vi "Enabled Channel Mask To Number.vi"(0 "selected acquisition channels to store":bool[](array[boolean])) -> (4 "number of selected channels":u8)   [LabVIEW 2021, in "Device Session.lvclass"]
uses:
  Device Session.lvclass
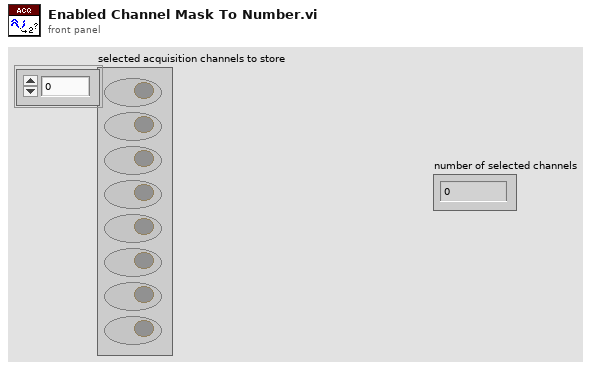
[diagram p1: front panel]
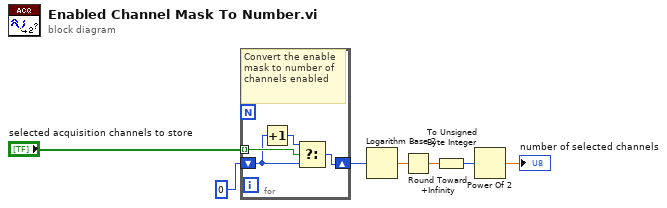
[diagram p0: block diagram]
diagram:
  n1 = for {
    tunnel: "selected acquisition channels to store" -> [w11] mode=indexing
    shift-right: [w9] -> w5
    shift-left: u8 0 -> [w8]
    # "Convert the enable mask to number of channels enabled"
    n2 = Increment(x=w8) -> (x+1=w10:u8)
    n3 = Select(t=w10, s=w11, f=w8) -> (s? t:f=w9:u8)
  }
  n4 = Logarithm Base 2(1:w5) -> (0:w4:dbl)
  n5 = Round Toward +Infinity(x=w4) -> (ceil(x): smallest int >= x=w3:dbl)
  n6 = To Unsigned Byte Integer(number=w3) -> (unsigned 8bit integer=w2:u8)
  n7 = Power Of 2(x=w2) -> (2^x=→"number of selected channels":dbl)
